vi "Read.vi"(0 "VISA resource name":refnum<visa-resource-name>, 5 "Single Lock-in Parameter (0: X output)":u16(ring) items=["X output", "Y output", "R output", "Theta output", "Aux In 1", "Aux In 2", "Aux In 3", "Aux In 4", "Aux Out 1", "Aux Out 2", "Xnoise", "Ynoise", "Reference Phase", "Sine Out Amplitude", "DC Level", "Int. Ref. Frequency", "Ext. Ref. Frequency"], 7 "Aux Input (1: Aux In 1)":u16(ring)=1 items=["Aux In 1"=1, "Aux In 2"=2, "Aux In 3"=3, "Aux In 4"=4], 9 "Data Channel (1: Data Channel 1(green))":i32(ring)=1 items=["Data Channel 1(green)"=1, "Data Channel 2(blue)"=2, "Data Channel 3(yellow)"=3, "Data Channel 4(orange)"=4], 11 "error in (no error)":errorcluster) -> (4 "VISA resource name out":refnum<visa-resource-name>, 6 "Single Lock-in Value":dbl format="%#_13f", 8 "Data Channel Value":dbl format="%#_13f", 10 "Aux Input Voltage":dbl format="%#_13f", 15 "error out":errorcluster)   [LabVIEW 2020, in "Stanford Research SR865.lvlib"]
doc: "Reads single parameter and returns single measurement from the instrument."
uses:
  Stanford Research SR865.lvlib
panel:
  # "Input Generator"
  # "Output"
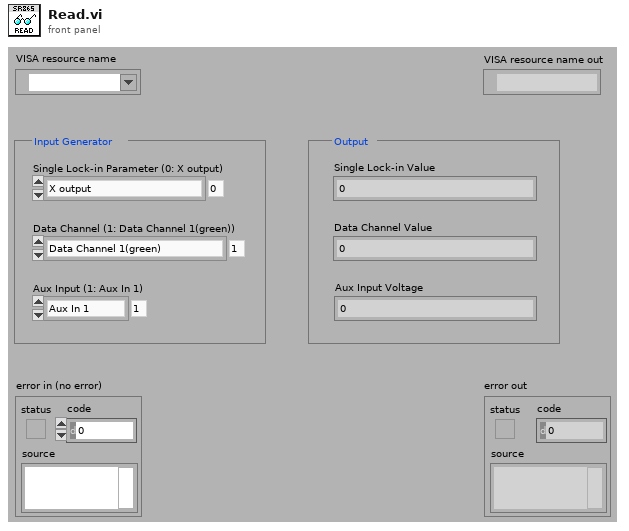
[diagram p1: front panel]
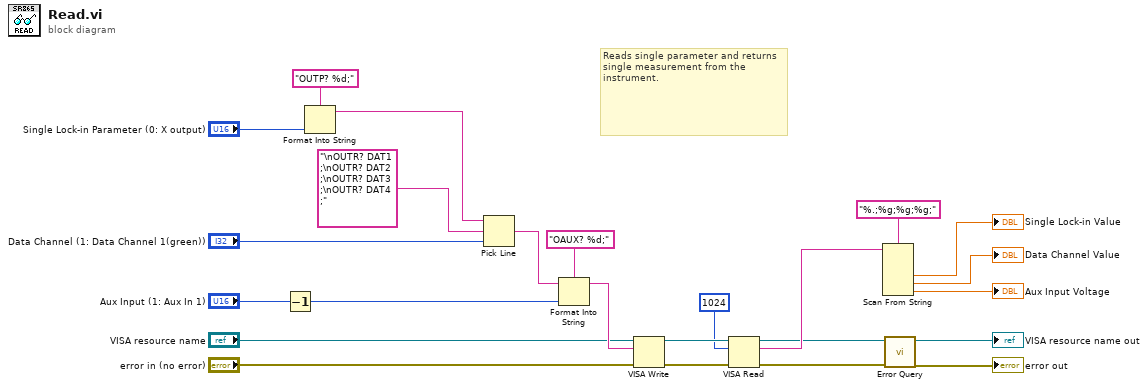
[diagram p0: block diagram]
diagram:
  # "Reads single parameter and returns single measurement from the instrument."
  n1 = Decrement(x="Aux Input (1: Aux In 1)") -> (x-1=w2:u16)
  n2 = Format Into String(format string="OUTP? %d;", "Single Lock-in Parameter (0: X output)") -> (resulting string=w20:string)  [unwired: 2 in, 1 out]
  n3 = Pick Line(string ("")=w20, multi-line string="\nOUTR? DAT1 ;\nOUTR? DAT2 ;\nOUTR? DAT3 ;\nOUTR? DAT4 ;", line index="Data Channel (1: Data Channel 1(green))") -> (output string=w19:string)
  n4 = Format Into String(format string="OAUX? %d;", initial string=w19, w2) -> (resulting string=w17:string)  [unwired: 1 in, 1 out]
  n5 = VISA Write(VISA resource name="VISA resource name", write buffer=w17, error in (no error)="error in (no error)") -> (VISA resource name out=w12:refnum<visa-resource-name>, error out=w11:errorcluster)  [unwired: 1 out]
  n6 = VISA Read(VISA resource name=w12, byte count=u32 1024, error in (no error)=w11) -> (VISA resource name out=w8:refnum<visa-resource-name>, read buffer=w9:string, error out=w7:errorcluster)  [unwired: 1 out]
  n7 = Scan From String(format string="%.;%g;%g;%g;", input string=w9) -> (output 1=→"Single Lock-in Value":dbl, output 2=→"Data Channel Value":dbl, output 3=→"Aux Input Voltage":dbl)  [unwired: 5 in, 3 out]
  n8 = call "Error Query.vi"("error in (no error)"=w7, "VISA resource name"=w8) -> ("error out"=→"error out":errorcluster, "VISA resource name out"=→"VISA resource name out":refnum<visa-resource-name>)  [unwired: 7 in, 1 out]
